vi "Process-error-listener.vi"(8 "error in (no error)":errorcluster, 11 "Errors in":T1) -> (0 "error out":errorcluster, 3 "Errors out":T1)   [LabVIEW 2013, in "Error-handling.lvlib" / "Errors.lvclass"]
uses:
  Errors.lvclass
  Object-reference.ctl
  Errors.lvclass/Errors.ctl
  Read Error event.vi
panel:
  in  "stop":bool
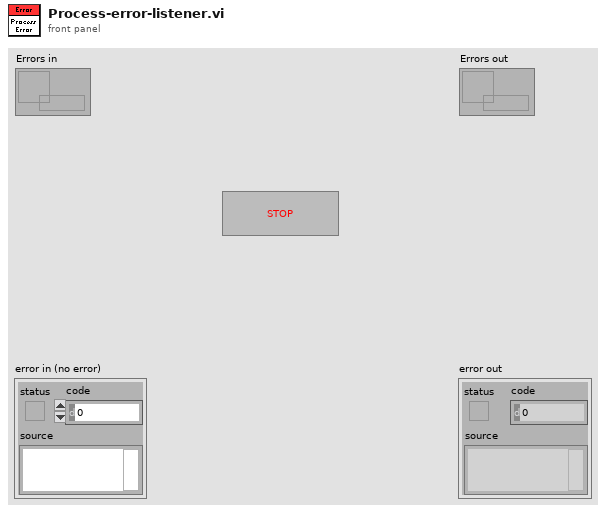
[diagram p1: front panel]
types:
  T1 = typedef "Error-handling.lvlib/Errors.lvclass/Object-reference.ctl" = refnum<data-value>
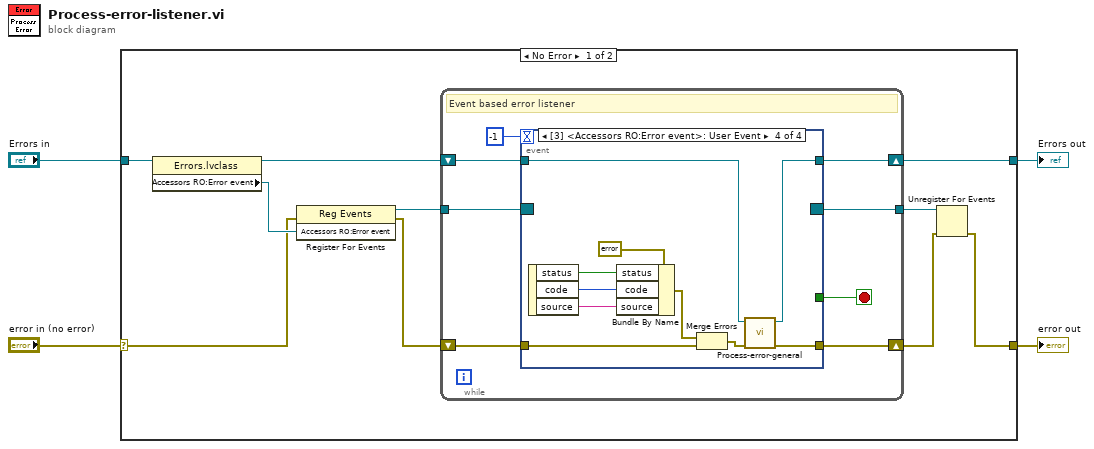
[diagram p0: block diagram]
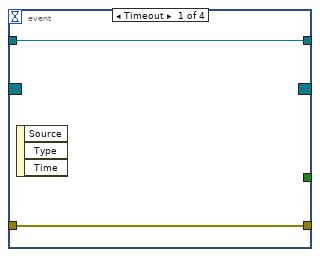
[diagram p2: hidden frame]
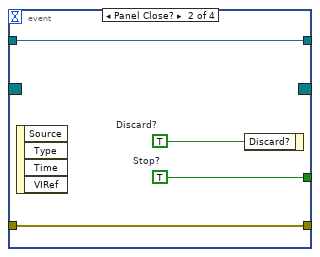
[diagram p3: hidden frame]
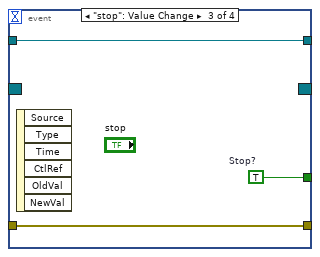
[diagram p4: hidden frame]
diagram:
  n1 = case shown="No Error" "error in (no error)" {
    selector: "error in (no error)" -> [w12 w42]
    tunnel: [w5 w42] -> w3
    tunnel: [w8 w43] -> w1
    tunnel: "Errors in" -> [w14 w43]
    frame No Error {
      n2 = property class="Errors.lvclass"(reference=w14) -> (reference out=w9:T1, "Accessors RO:Error event"=w13:refnum<user-event>)  [unwired: 1 in, 1 out]
      n3 = register-events(error in=w12, w13) -> (reference out=w11:refnum<event-registration>, error out=w10:errorcluster)  [unwired: 1 in]
      n4 = while {
        tunnel: w11 -> [w22]
        shift-right: [w20] -> w6
        shift-left: w10 -> [w21]
        shift-right: [w16] -> w8
        shift-left: w9 -> [w17]
        tunnel: [w15] -> w7
        stop <- w19 stop-if-true
        # "Event based error listener"
        n5 = event shown="[3] <Accessors RO:Error event>: User Event" {
          selector: w22 -> [_ _ _ _]
          dyn-events: [_ _ _ _] -> w15
          timeout: -1 -> [_ _ _ _]
          tunnel: w21 -> [w24 w26 w31 w36]
          tunnel: [w24 w26 w31 w34] -> w20
          tunnel: [_ w27 w30 _] -> w19
          tunnel: w17 -> [w23 w25 w29 w33]
          tunnel: [w23 w25 w29 w32] -> w16
          event Timeout {
            n6 = event-data() -> ()  [unwired: 1 in, 3 out]
          }
          event Panel Close? {
            w27 = TRUE  # Stop?
            w28 = TRUE  # Discard?
            n7 = event-data() -> ()  [unwired: 1 in, 4 out]
            n8 = event-data("Discard?"=w28) -> ()  [unwired: 1 in, 1 out]
          }
          event "stop": Value Change {
            w30 = TRUE  # Stop?
            n9 = event-data() -> ()  [unwired: 1 in, 6 out]
          }
          event User Event {
            n10 = event-data() -> ("status"=w40:bool, "code"=w39:i32, "source"=w38:string)  [unwired: 1 in]
            n11 = Bundle By Name(cluster=errorcluster {"status"=FALSE, "code"=0, "source"=""} ("error constant"), "status"=w40, "code"=w39, "source"=w38) -> (w37:errorcluster)
            n12 = Merge Errors(w37, w36) -> (w35:errorcluster)
            n13 = call "Process-error-general.vi"("error in (no error)"=w35, "Errors in"=w33) -> ("error out"=w34:errorcluster, "Errors out"=w32:T1)  [unwired: 8 in]
          }
        }
      }
      n14 = Unregister For Events(event registration refnum=w7, error in=w6) -> (error out=w5:errorcluster)
    }
    frame Error {
    }
  }
  "error out" <- w3
  "Errors out" <- w1
